vi "CoffeeMachine.vi"() -> ()   [LabVIEW 2020]
uses:
  Typedefs/Operations.ctl
  Typedefs/CoffeeMachineData.ctl
  <vilib>/Utility/config.llb/Config Data RefNum.ctl
  <vilib>/Utility/config.llb/Read Key (I32).vi
  <vilib>/Utility/config.llb/NI_LVConfig.lvlib
panel:
  out "No. of Cups":dbl
  out "Array":i32[](array[numeric])
  out "keys":string[](array[string])
  out "section names":string[](array[string])
  out "Dsipensing":bool
  out "Brewing":bool
  out "Grinding":bool
  out "Heating":bool
  out "Purging":bool
  out "Low Milk":bool
  out "Low Bean":bool
  out "Low Water":bool
  out "Total Cups":dbl
  out "Elapsed Time":i32
  in  "Power":bool
  out "Dispenser":dbl(slide) scale=0.0..60.0
  out "Chamber":dbl(slide) scale=0.0..60.0
  in  "Milk Level":dbl(slide) scale=0.0..100.0
  in  "Bean Level":dbl(slide) scale=0.0..100.0
  in  "Water Level":dbl(slide) scale=0.0..100.0
  in  "Type":u8(knob) scale=0.0..2.0
  in  "1 Carafe":bool
  in  "1 Cup":bool
  in  "Error in (no error)":errorcluster
  out "Error Out":errorcluster
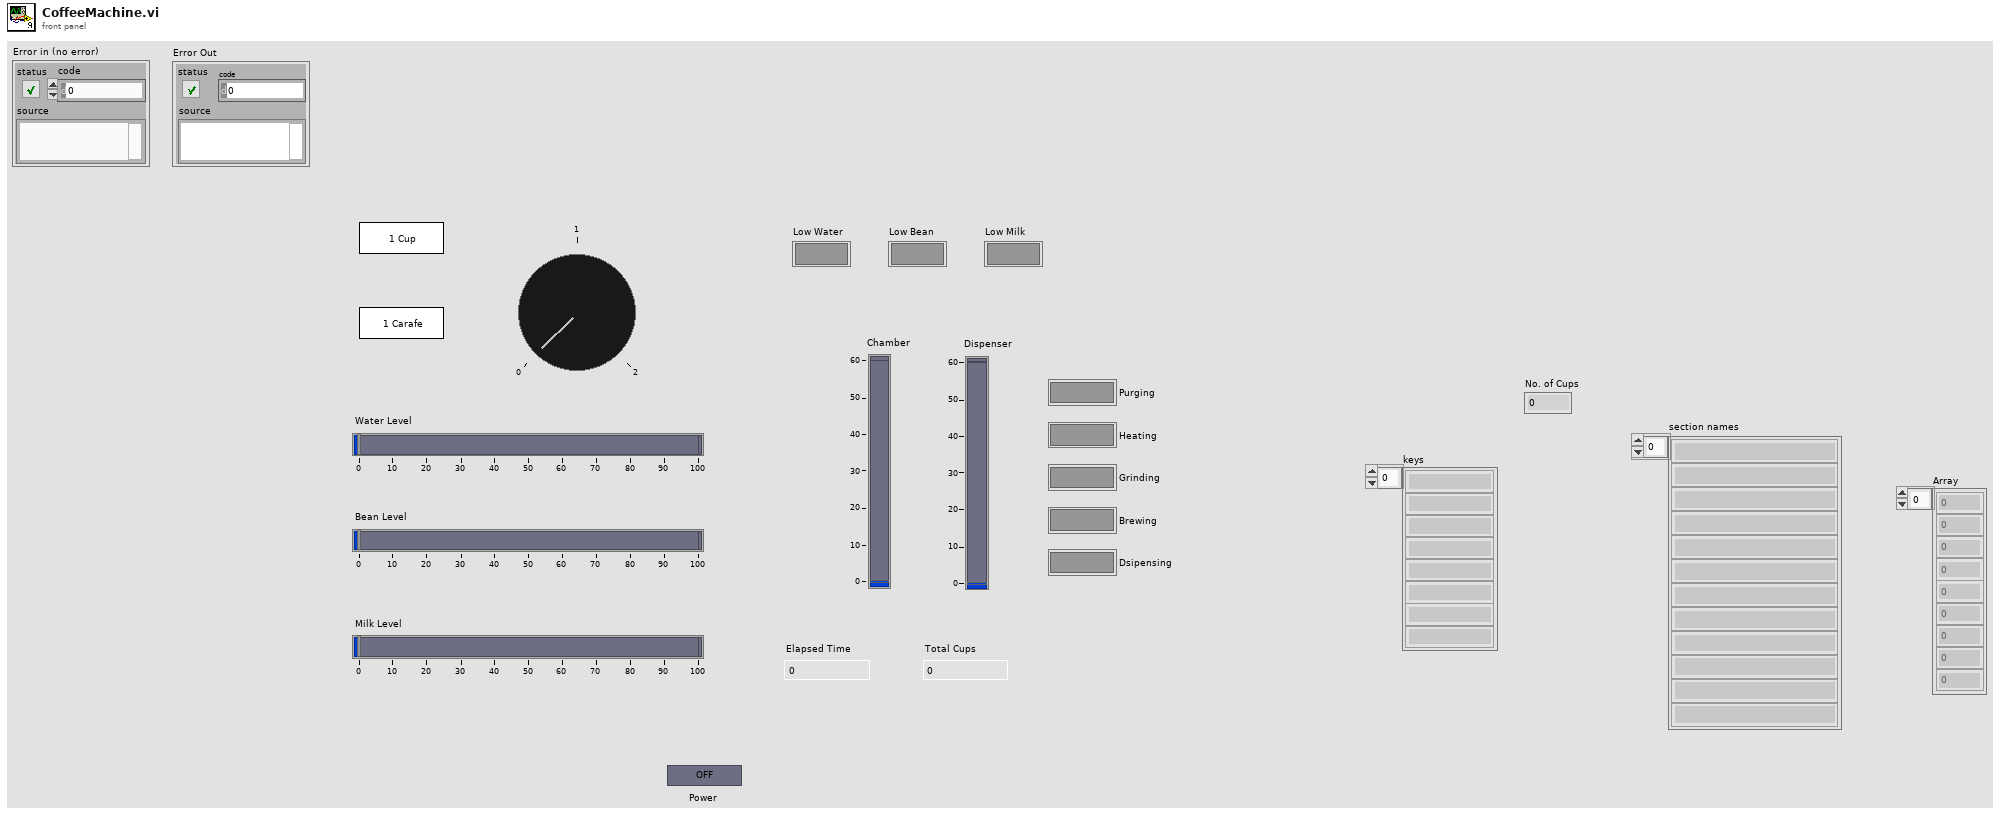
[diagram p1: front panel]
types:
  T1 = typedef "CoffeeMachineData.ctl" = cluster{"Power":bool, "1 Cup":bool, "1 Carafe":bool, "Type":u8, "Water Level":dbl, "Bean Level":dbl, "Milk Level":dbl, "Low Water":bool, "Low Bean":bool, "Low Milk":bool, "Chamber":dbl, "Dispenser":dbl, "Purging":bool, "Heating":bool, "Grinding":bool, "Brewing":bool, "Dispensing":bool, "Elapsed Time":dbl, "Total Cups":dbl, "Start Time":dbl, "File Path":path, "Sufficient Ingredients":bool, "File Reference":T2, "Section Array":string[], "Key Array":string[], "Values Array":i32[], "Section Count":dbl, "Required Section":string, "Type Chosen":bool, "No. of Cups":dbl, "No of Cups Selected":bool}
  T2 = typedef "NI_LVConfig.lvlib/Config Data RefNum.ctl" = refnum<k1>
  T3 = typedef "Operations.ctl" = enum16{"Create Q", "Enqueue 1", "Enqueue N", "Enstack 1", "Dequeue", "Flush Q", "Release Q"}
  T4 = enum8{"Enabled", "Disabled", "Disabled and Grayed Out"}
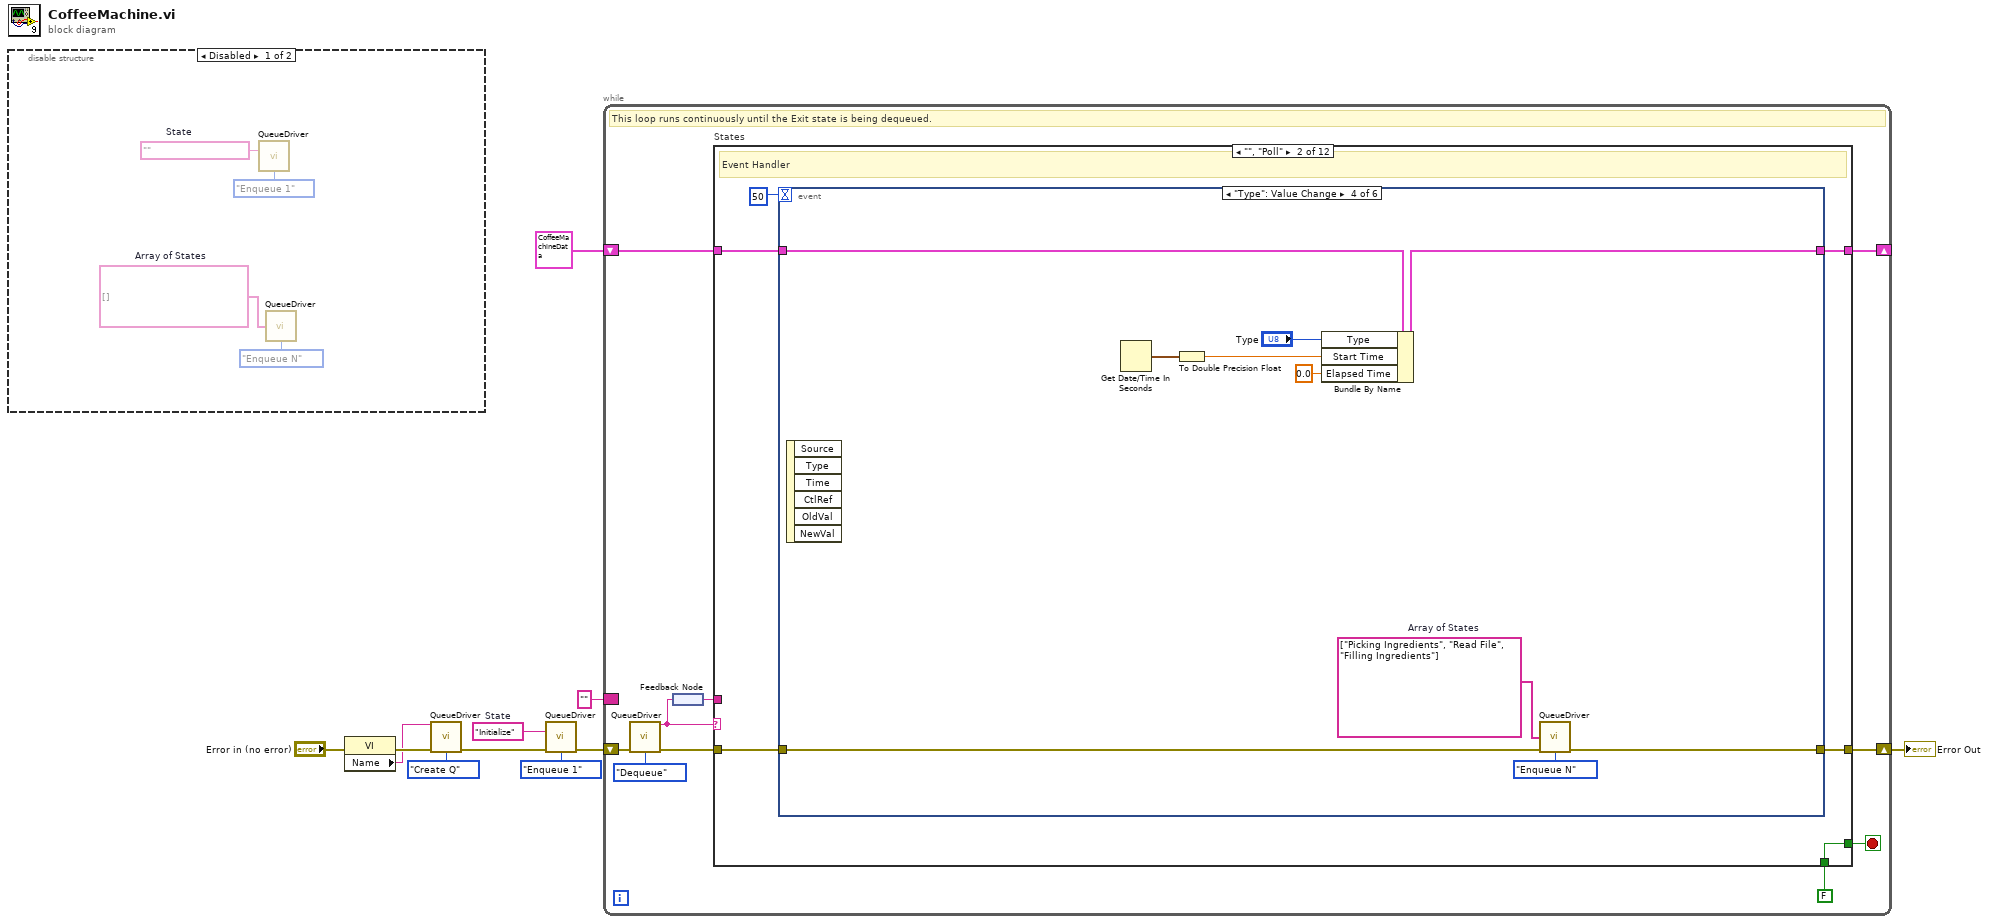
[diagram p0: block diagram]
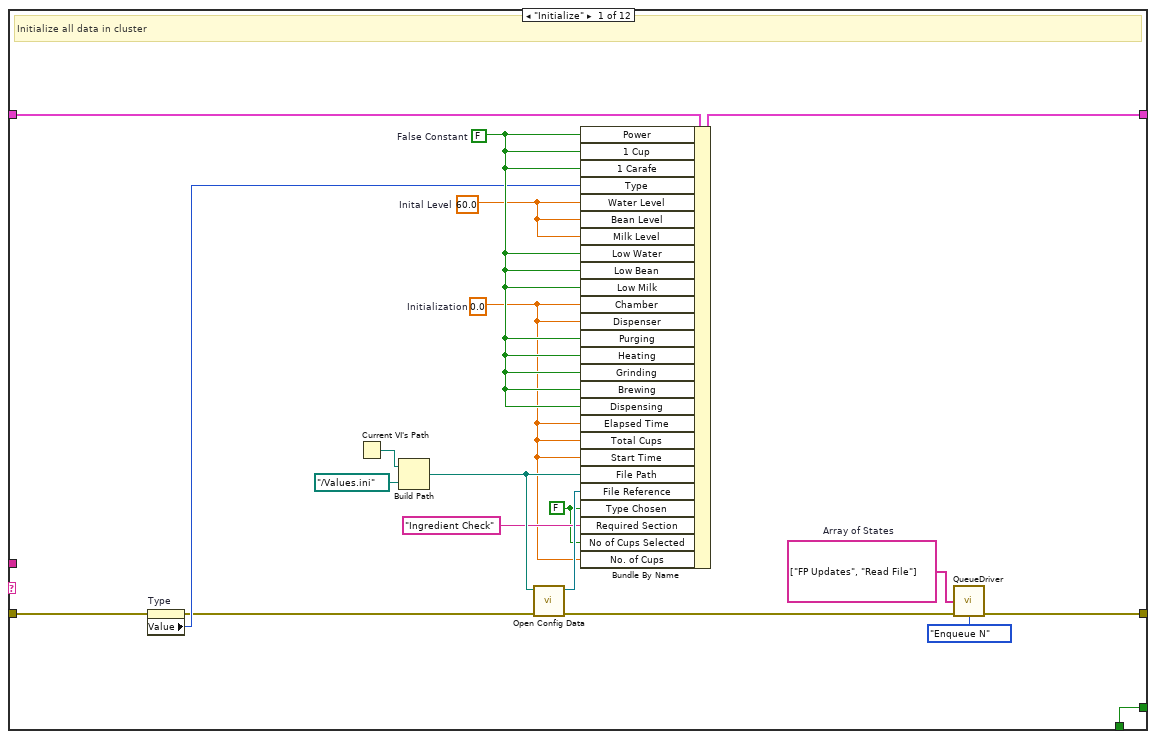
[diagram p3: hidden frame]
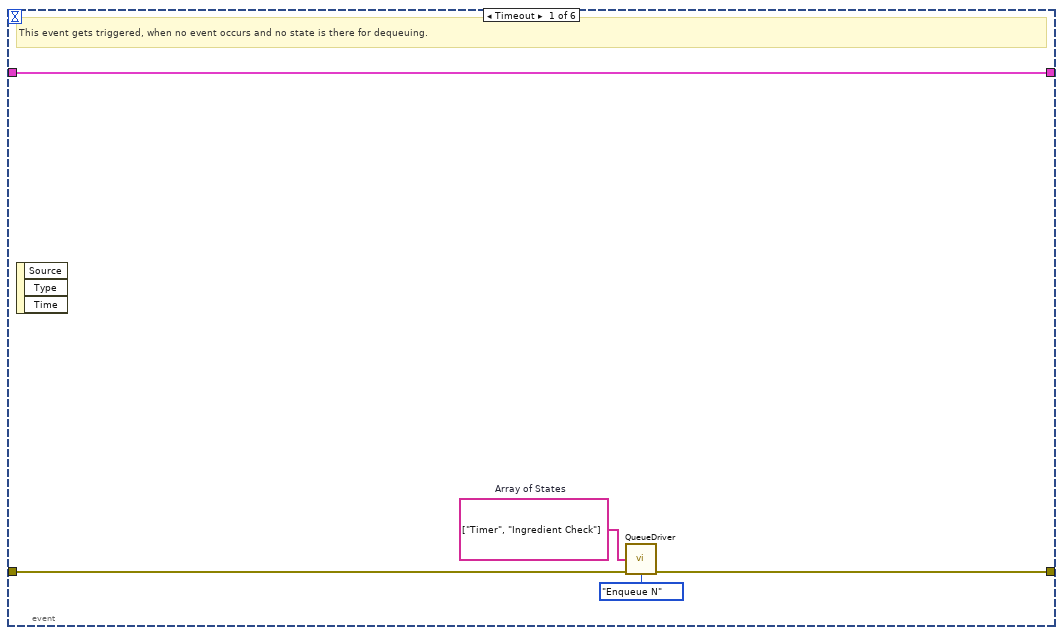
[diagram p4: hidden frame]
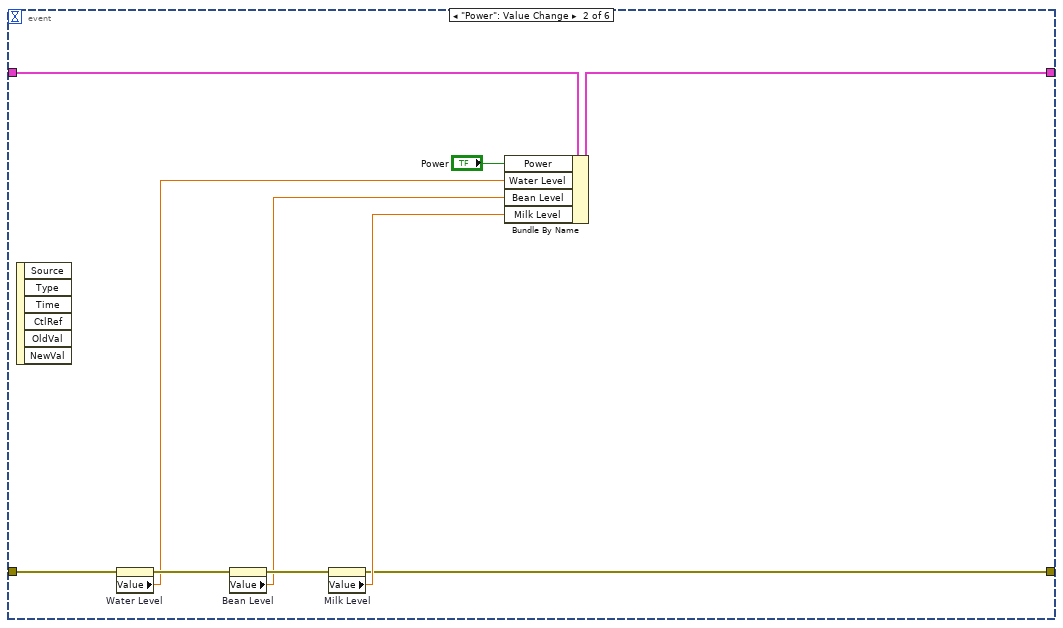
[diagram p5: hidden frame]
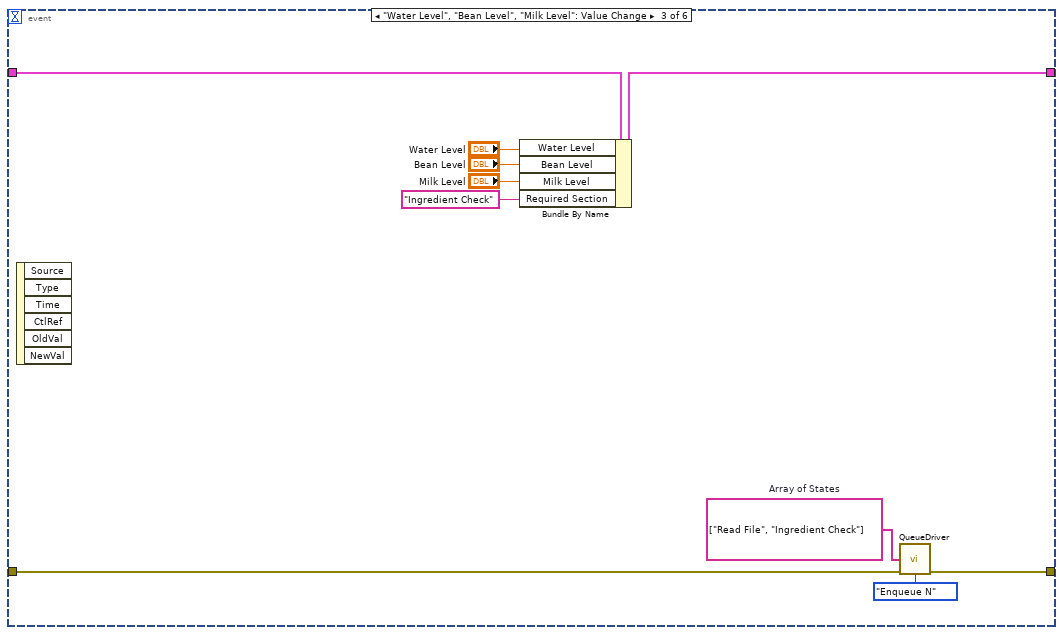
[diagram p6: hidden frame]
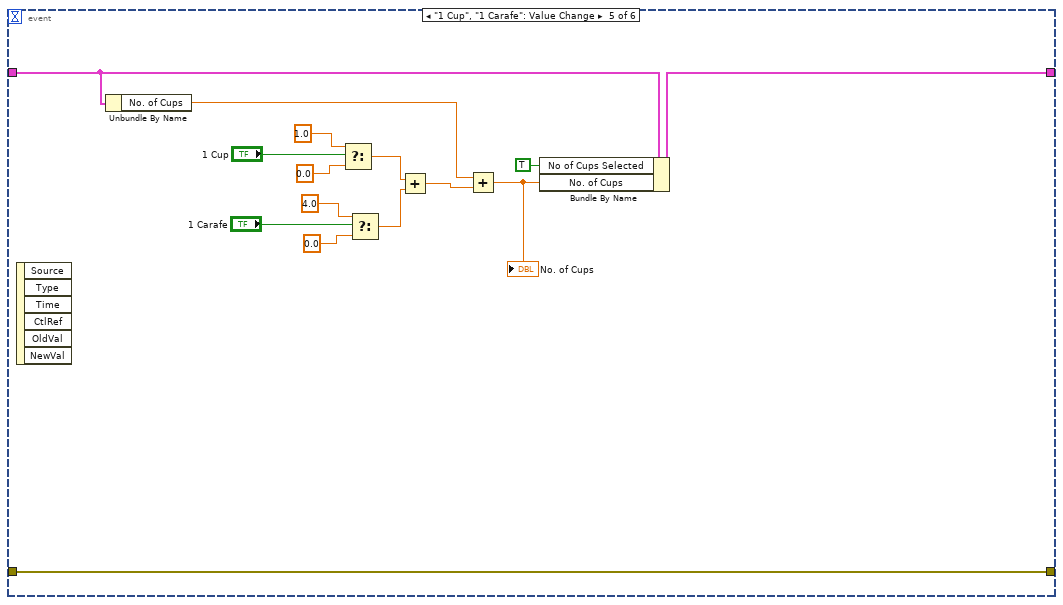
[diagram p7: hidden frame]
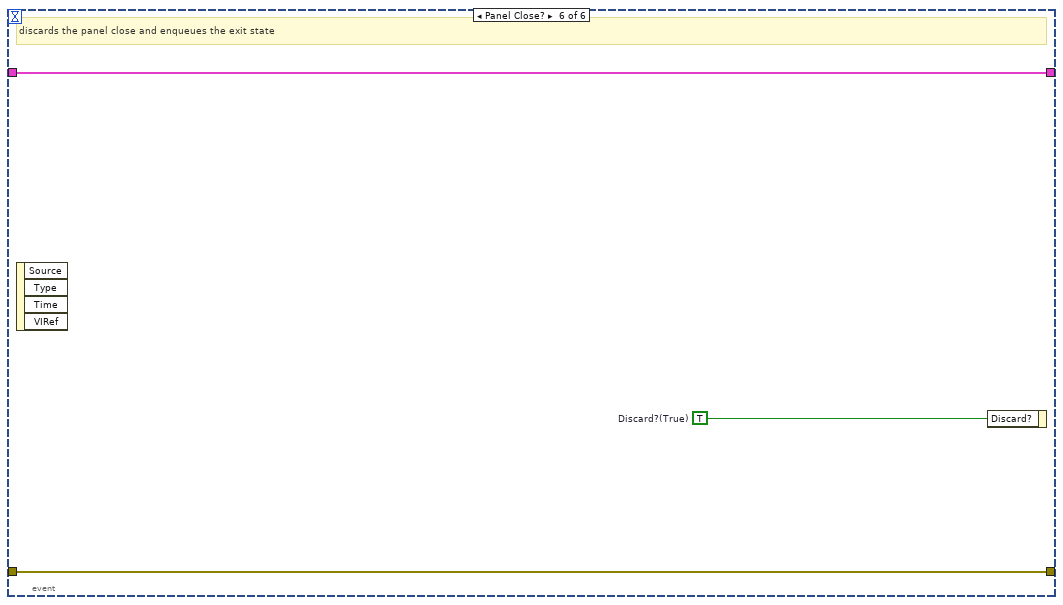
[diagram p8: hidden frame]
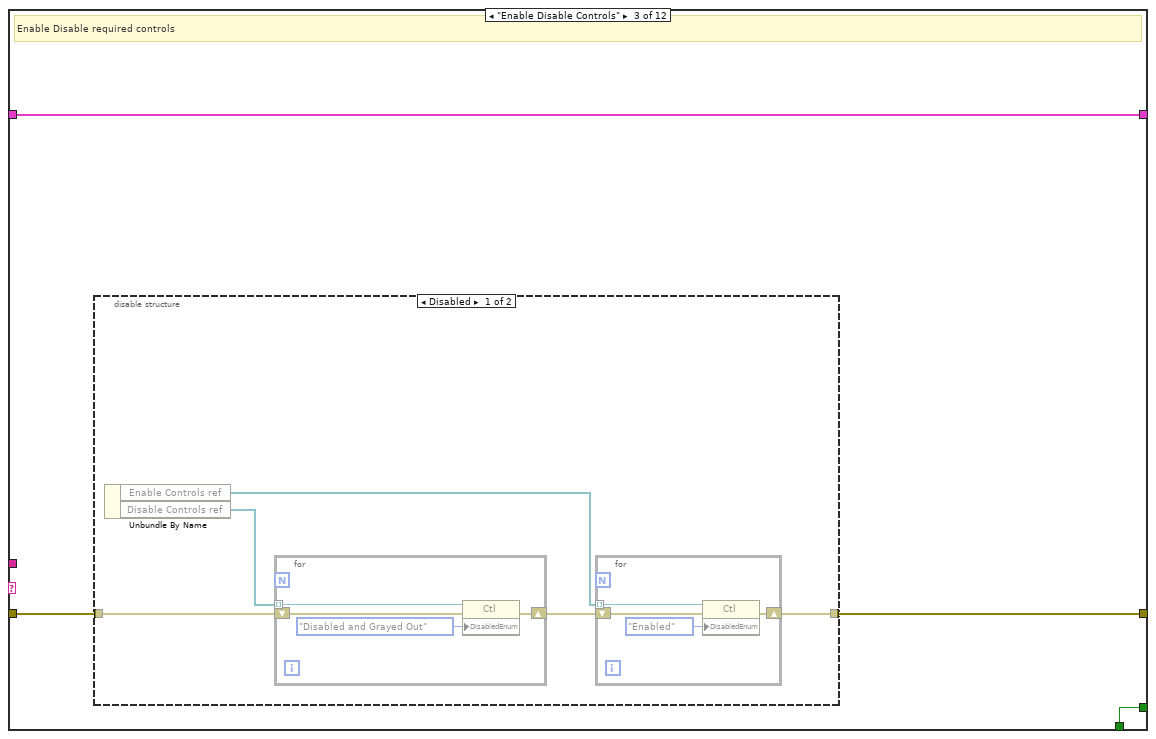
[diagram p9: hidden frame]
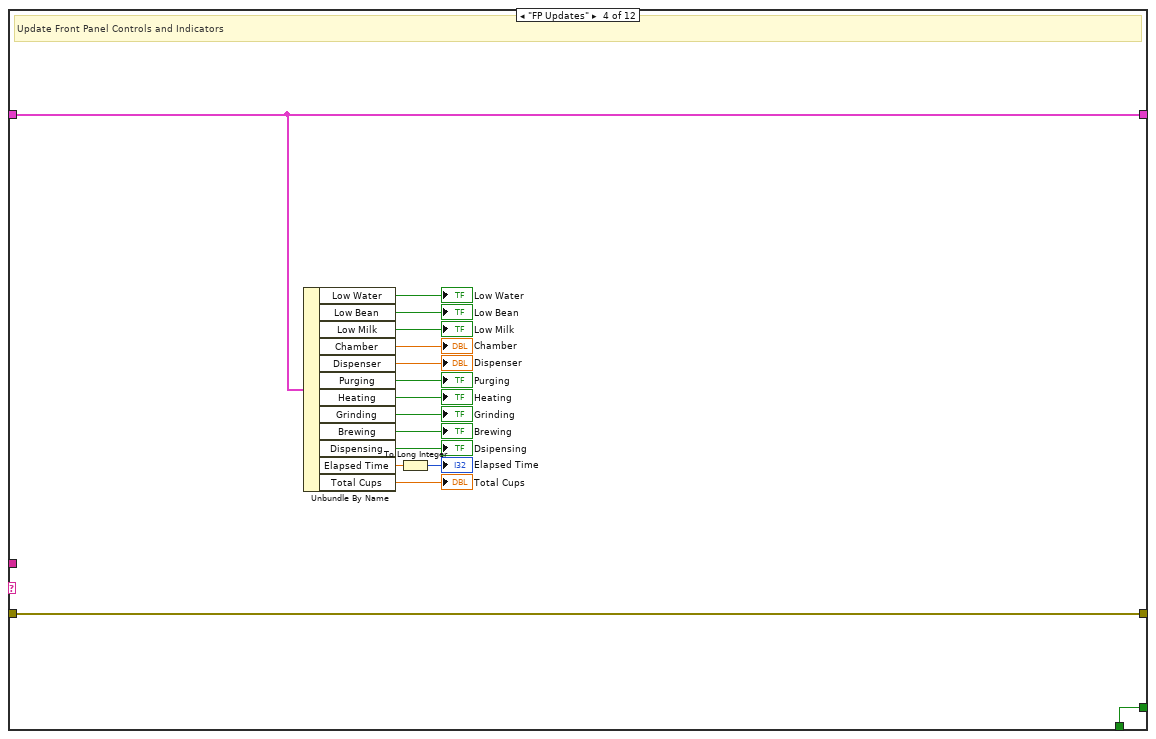
[diagram p11: hidden frame]
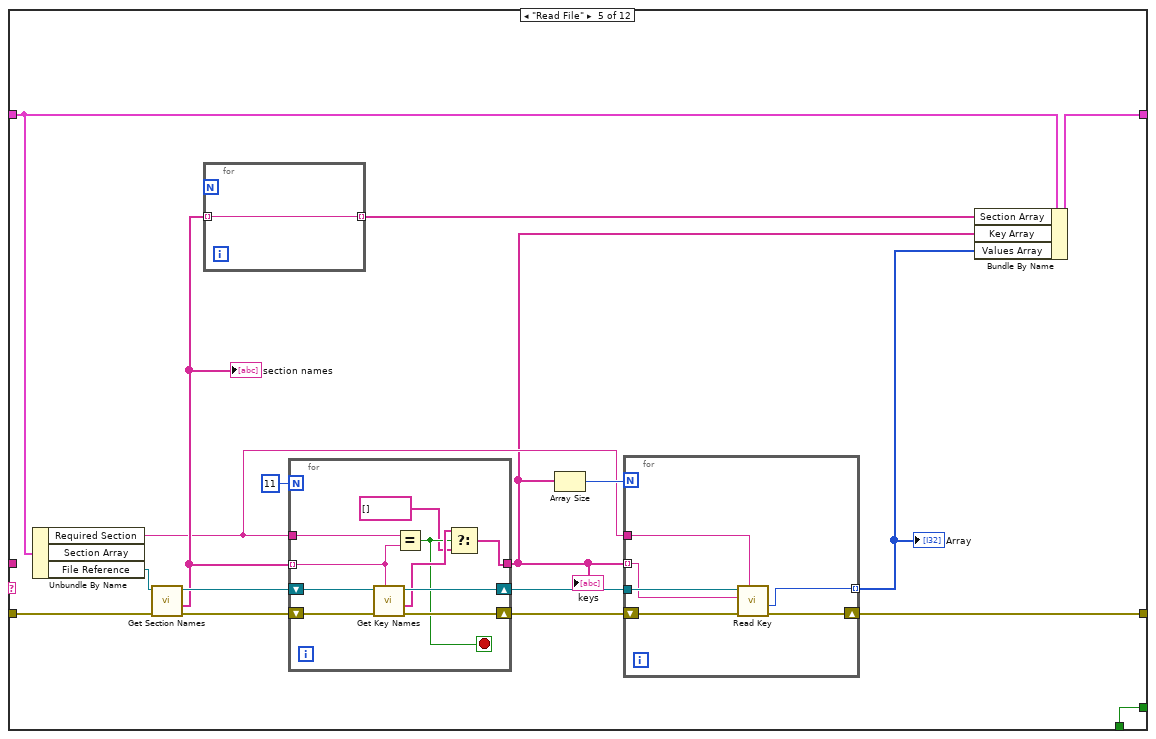
[diagram p12: hidden frame]
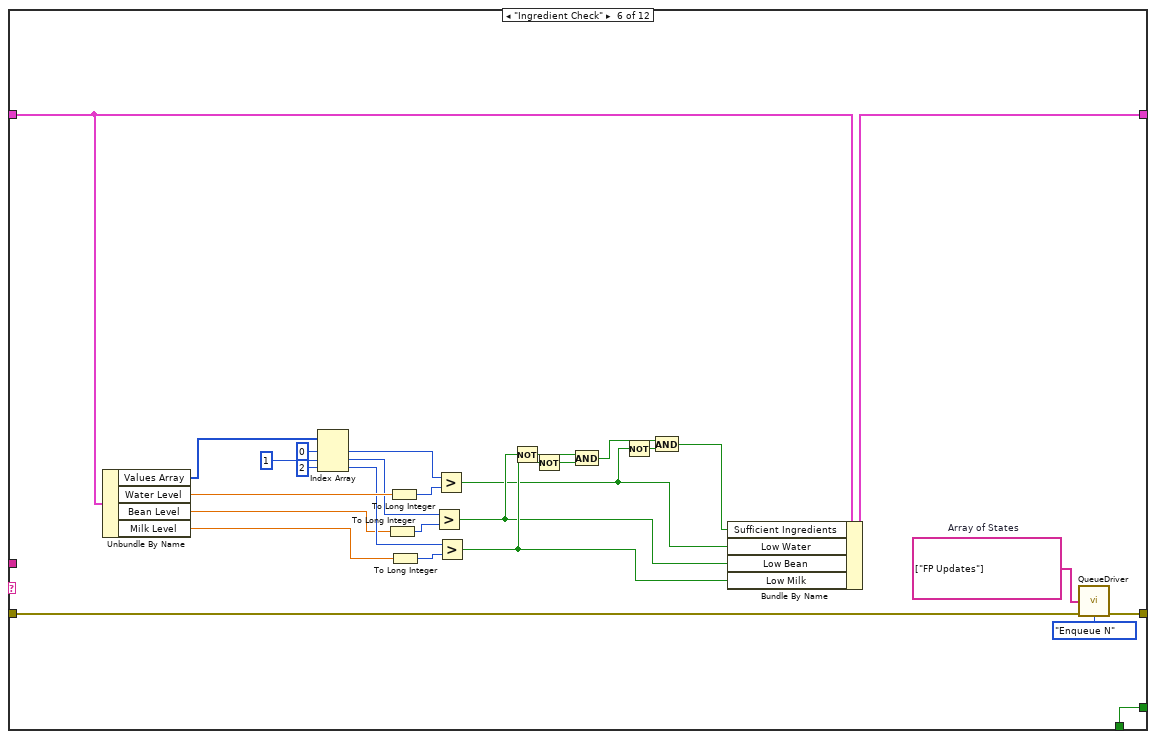
[diagram p13: hidden frame]
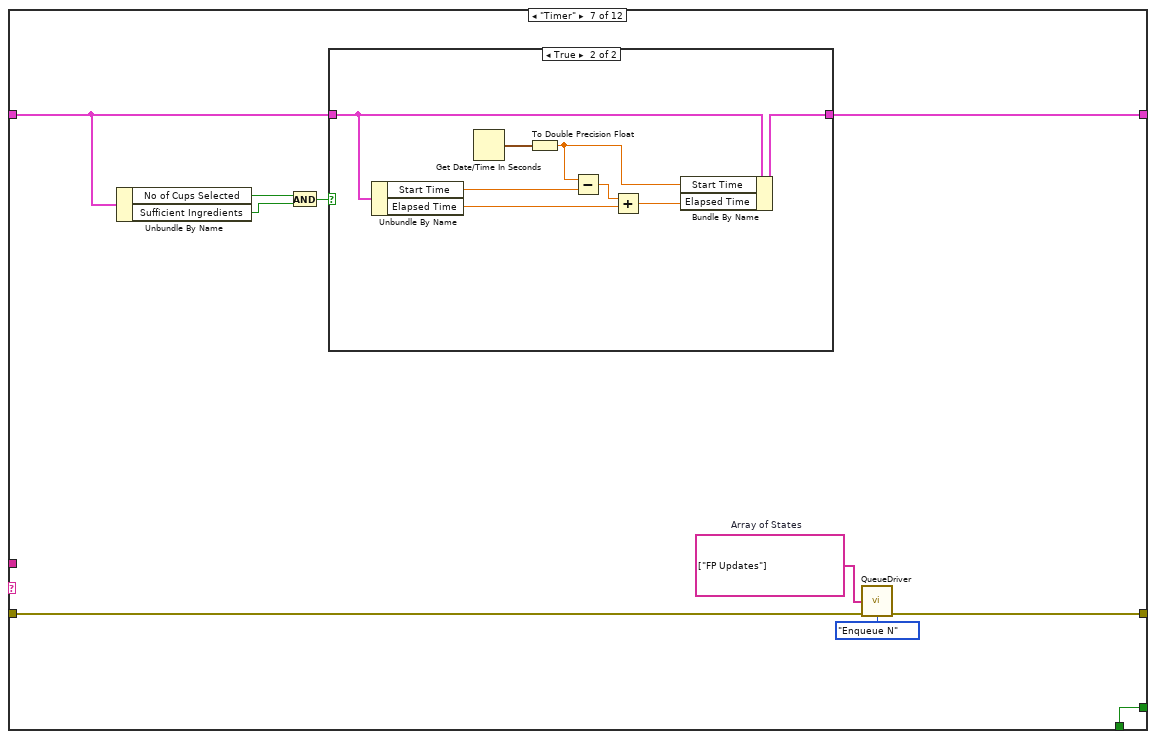
[diagram p14: hidden frame]
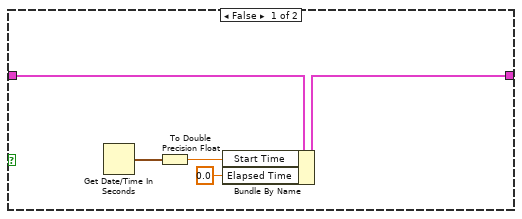
[diagram p15: hidden frame]
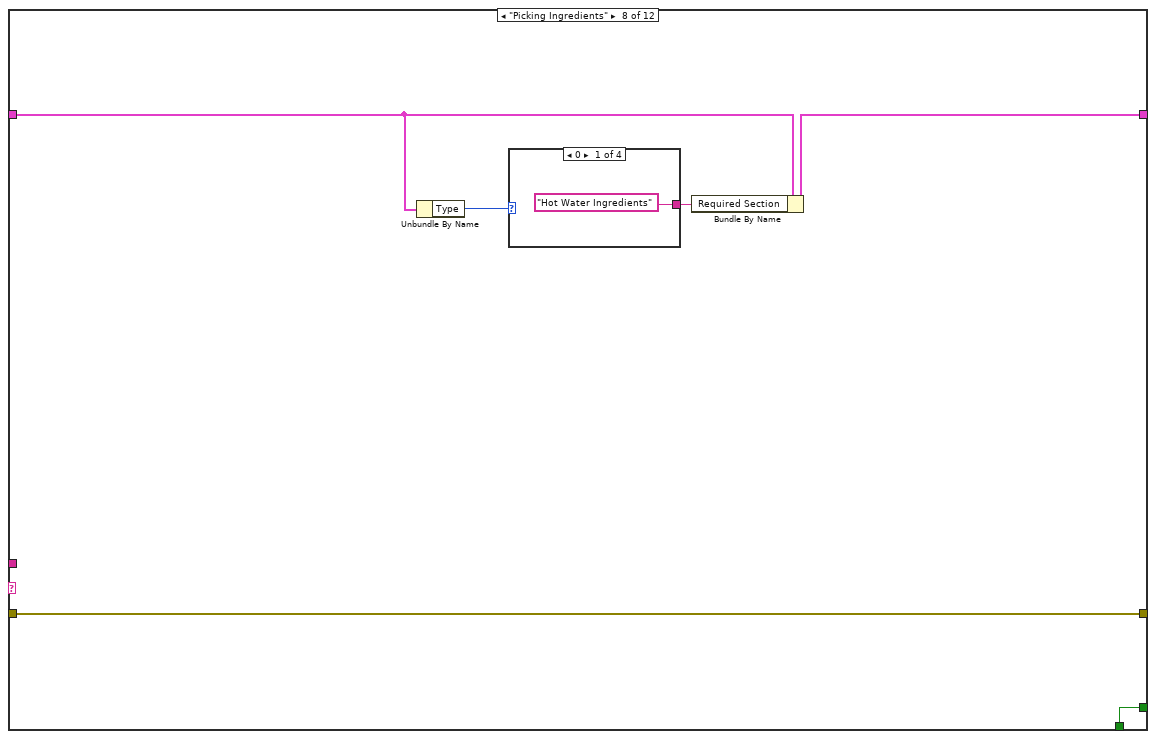
[diagram p16: hidden frame]
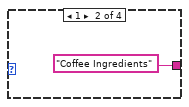
[diagram p17: hidden frame]
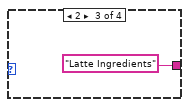
[diagram p18: hidden frame]
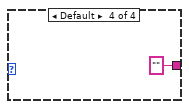
[diagram p19: hidden frame]
diagram:
  w6 = "Initialize"  # State
  n1 = disable-structure shown="Disabled" {
    frame Disabled {
      w12 = string[] []  # Array of States
      w14 = ""  # State
      n2 = call "QueueDriver.vi"("State"=w14, "Operations"=Operations."Enqueue 1" ("Queue Operations")) -> ()  [unwired: 12 in, 2 out]
      n3 = call "QueueDriver.vi"("Array of States"=w12, "Operations"=Operations."Enqueue N" ("Queue Operations")) -> ()  [unwired: 12 in, 2 out]
    }
    frame Enabled {
    }
  }
  n4 = property class="VI"(error in="Error in (no error)") -> (error out=w7:errorcluster, "Name"=w2:string)  [unwired: 1 in, 1 out]
  n5 = call "QueueDriver.vi"("Queue Name"=w2, "error in (no error)"=w7, "Operations"=Operations."Create Q" ("Queue Operations")) -> ("error out"=w3:errorcluster)  [unwired: 11 in, 1 out]
  n6 = call "QueueDriver.vi"("State"=w6, "error in (no error)"=w3, "Operations"=Operations."Enqueue 1" ("Queue Operations")) -> ("error out"=w4:errorcluster)  [unwired: 11 in, 1 out]
  n7 = while {
    border: "" ("States[]") -> [_]
    shift-right: [w24] -> w10
    shift-left: w4 -> [w19]
    shift-right: [w16] -> _
    shift-left: T1 {"Power"=FALSE, "1 Cup"=FALSE, "1 Carafe"=FALSE, "Type"=0, "Water Level"=0.0, "Bean Level"=0.0, "Milk Level"=0.0, "Low Water"=FALSE, "Low Bean"=FALSE, "Low Milk"=FALSE, "Chamber"=0.0, "Dispenser"=0.0, "Purging"=FALSE, "Heating"=FALSE, "Grinding"=FALSE, "Brewing"=FALSE, "Dispensing"=FALSE, "Elapsed Time"=0.0, "Total Cups"=0.0, "Start Time"=0.0, "File Path"=path "", "Sufficient Ingredients"=FALSE, "File Reference"=refnum, "Section Array"=[], "Key Array"=[], "Values Array"=[], "Section Count"=0.0, "Required Section"="", "Type Chosen"=FALSE, "No. of Cups"=0.0, "No of Cups Selected"=FALSE} -> [w17]
    stop <- w23 stop-if-true
    # "This loop runs continuously until the Exit state is being dequeued."
    n8 = call "QueueDriver.vi"("error in (no error)"=w19, "Operations"=Operations."Dequeue" ("Queue Operations")) -> ("Dequeued State"=w18:string, "error out"=w20:errorcluster)  [unwired: 12 in]
    n9 = feedback #1() -> (w25:string)
    n10 = feedback-in #1(w18) -> ()
    n11 = case "States" shown="\"\", \"Poll\"" w18 {
      selector: w18 -> [_ _ _ _ _ _ _ _ _ _ w258 _]
      tunnel: w20 -> [w37 w50 w107 w136 w150 w197 w203 w226 w232 w241 w262 w280]
      tunnel: w25 -> [_ _ _ _ _ _ _ _ _ w240 _ _]
      tunnel: [w29 w49 w106 w136 w147 w192 w202 w226 w232 w237 w259 w278] -> w24
      tunnel: FALSE -> [w44 w48 w105 w135 w153 w191 w206 w227 w234 w236 w257 _]
      tunnel: [w44 w48 w105 w135 w153 w191 w206 w227 w234 w236 w257 TRUE] -> w23
      tunnel: w17 -> [w43 w45 w104 w134 w152 w198 w208 w225 w233 w235 w256 w277]
      tunnel: [w42 w46 w104 w134 w146 w195 w207 w223 w233 w235 w256 w277] -> w16
      frame "Initialize" {
        w27 = FALSE ("Type Chosen")
        w32 = string[] ["FP Updates", "Read File"]  # Array of States
        w26 = 0.0  # Initialization
        w38 = 60.0  # Inital Level
        w39 = FALSE  # False Constant
        # "Initialize all data in cluster"
        n12 = property on="Type" class="Knob (strict)"(error in=w37) -> (error out=w35:errorcluster, "Value"=w36:u8)  [unwired: 1 in, 1 out]
        n13 = Current VI's Path() -> (path=w41:path)
        n14 = Build Path(base path=w41, name or relative path=path "../Values.ini") -> (appended path=w34:path)
        n15 = call <vilib>:"Open Config Data.vi"("error in (no error)"=w35, "configuration file path"=w34) -> ("error out"=w30:errorcluster, "refnum"=w33:T2)  [unwired: 7 in, 1 out]
        n16 = Bundle By Name(cluster=w43, "Power"=w39, "1 Cup"=w39, "1 Carafe"=w39, "Type"=w36, "Water Level"=w38, "Bean Level"=w38, "Milk Level"=w38, "Low Water"=w39, "Low Bean"=w39, "Low Milk"=w39, "Chamber"=w26, "Dispenser"=w26, "Purging"=w39, "Heating"=w39, "Grinding"=w39, "Brewing"=w39, "Dispensing"=w39, "Elapsed Time"=w26, "Total Cups"=w26, "Start Time"=w26, "File Path"=w34, "File Reference"=w33, "Type Chosen"=w27, "Required Section"="Ingredient Check", "No of Cups Selected"=w27, "No. of Cups"=w26) -> (w42:T1)
        n17 = call "QueueDriver.vi"("Array of States"=w32, "error in (no error)"=w30, "Operations"=Operations."Enqueue N" ("Queue Operations")) -> ("error out"=w29:errorcluster)  [unwired: 11 in, 1 out]
      }
      frame "", "Poll" {
        # "Event Handler"
        n18 = event shown="[3] \"Type\": Value Change" {
          selector: _ -> [_ _ _ _ _ _]
          dyn-events: _ -> [_ _ _ _ _ _]
          timeout: 50 -> [_ _ _ _ _ _]
          tunnel: w50 -> [w52 w62 w67 w78 w100 w103]
          tunnel: [w51 w56 w66 w77 w100 w103] -> w49
          tunnel: [w55 w64 w74 w84 w96 w101] -> w46
          tunnel: w45 -> [w55 w65 w75 w85 w89 w101]
          event Timeout {
            w54 = string[] ["Timer", "Ingredient Check"]  # Array of States
            # "This event gets triggered, when no event occurs and no state is there for dequeuing."
            n19 = event-data() -> ()  [unwired: 1 in, 3 out]
            n20 = call "QueueDriver.vi"("Array of States"=w54, "error in (no error)"=w52, "Operations"=Operations."Enqueue N" ("Queue Operations")) -> ("error out"=w51:errorcluster)  [unwired: 11 in, 1 out]
          }
          event "Power": Value Change {
            n21 = event-data() -> ()  [unwired: 1 in, 6 out]
            n22 = property on="Water Level" class="Slide (strict)"(error in=w62) -> (error out=w61:errorcluster, "Value"=w59:dbl)  [unwired: 1 in, 1 out]
            n23 = property on="Bean Level" class="Slide (strict)"(error in=w61) -> (error out=w60:errorcluster, "Value"=w58:dbl)  [unwired: 1 in, 1 out]
            n24 = property on="Milk Level" class="Slide (strict)"(error in=w60) -> (error out=w56:errorcluster, "Value"=w57:dbl)  [unwired: 1 in, 1 out]
            n25 = Bundle By Name(cluster=w65, "Power"="Power", "Water Level"=w59, "Bean Level"=w58, "Milk Level"=w57) -> (w64:T1)
          }
          event "Water Level", "Bean Level", "Milk Level": Value Change {
            w69 = string[] ["Read File", "Ingredient Check"]  # Array of States
            n26 = event-data() -> ()  [unwired: 1 in, 6 out]
            n27 = Bundle By Name(cluster=w75, "Water Level"="Water Level", "Bean Level"="Bean Level", "Milk Level"="Milk Level", "Required Section"="Ingredient Check") -> (w74:T1)
            n28 = call "QueueDriver.vi"("Array of States"=w69, "error in (no error)"=w67, "Operations"=Operations."Enqueue N" ("Queue Operations")) -> ("error out"=w66:errorcluster)  [unwired: 11 in, 1 out]
          }
          event "Type": Value Change {
            w80 = string[] ["Picking Ingredients", "Read File", "Filling Ingredients"]  # Array of States
            n29 = event-data() -> ()  [unwired: 1 in, 6 out]
            n30 = Get Date/Time In Seconds() -> (seconds since 1Jan1904=w82:timestamp)
            n31 = To Double Precision Float(number=w82) -> (double precision float=w81:dbl)
            n32 = Bundle By Name(cluster=w85, "Type"="Type", "Start Time"=w81, "Elapsed Time"=0.0) -> (w84:T1)
            n33 = call "QueueDriver.vi"("Array of States"=w80, "error in (no error)"=w78, "Operations"=Operations."Enqueue N" ("Queue Operations")) -> ("error out"=w77:errorcluster)  [unwired: 11 in, 1 out]
          }
          event "1 Cup", "1 Carafe": Value Change {
            n34 = event-data() -> ()  [unwired: 1 in, 6 out]
            n35 = Unbundle By Name(w89) -> ("No. of Cups"=w88:dbl)
            n36 = Select(t=1.0, s="1 Cup", f=0.0) -> (s? t:f=w91:dbl)
            n37 = Select(t=4.0, s="1 Carafe", f=0.0) -> (s? t:f=w90:dbl)
            n38 = Add(x=w91, y=w90) -> (x+y=w86:dbl)
            n39 = Add(x=w88, y=w86) -> (x+y=w87:dbl)
            "No. of Cups" <- w87
            n40 = Bundle By Name(cluster=w89, "No of Cups Selected"=TRUE, "No. of Cups"=w87) -> (w96:T1)
          }
          event Panel Close? {
            w102 = TRUE  # Discard?(True)
            # "discards the panel close and enqueues the exit state"
            n41 = event-data() -> ()  [unwired: 1 in, 4 out]
            n42 = event-data("Discard?"=w102) -> ()  [unwired: 1 in, 1 out]
          }
        }
      }
      frame "Enable Disable Controls" {
        # "Enable Disable required controls"
        n43 = disable-structure shown="Disabled" {
          disable-tunnel: w107 -> [w112 _]
          disable-tunnel: [w108 _] -> w106
          frame Disabled {
            n44 = Unbundle By Name() -> ("Enable Controls ref"=w109:refnum<vi>[], "Disable Controls ref"=w111:refnum<vi>[])  [unwired: 1 in]
            n45 = for {
              shift-right: [w119] -> w110
              shift-left: w112 -> [w120]
              tunnel: w111 -> [w117] mode=indexing
              n46 = property class="Ctl"(reference=w117, error in=w120, "DisabledEnum"=T4."Disabled and Grayed Out" ("Disabled")) -> (error out=w119:errorcluster)  [unwired: 1 out]
            }
            n47 = for {
              shift-right: [w115] -> w108
              shift-left: w110 -> [w116]
              tunnel: w109 -> [w113] mode=indexing
              n48 = property class="Ctl"(reference=w113, error in=w116, "DisabledEnum"=T4."Enabled" ("Disabled")) -> (error out=w115:errorcluster)  [unwired: 1 out]
            }
          }
          frame Enabled {
          }
        }
      }
      frame "FP Updates" {
        # "Update Front Panel Controls and Indicators"
        n49 = Unbundle By Name(w134) -> ("Low Water"=→"Low Water":bool, "Low Bean"=→"Low Bean":bool, "Low Milk"=→"Low Milk":bool, "Chamber"=→"Chamber":dbl, "Dispenser"=→"Dispenser":dbl, "Purging"=→"Purging":bool, "Heating"=→"Heating":bool, "Grinding"=→"Grinding":bool, "Brewing"=→"Brewing":bool, "Dispensing"=→"Dsipensing":bool, "Elapsed Time"=w123:dbl, "Total Cups"=→"Total Cups":dbl)
        n50 = To Long Integer(number=w123) -> (32bit integer=→"Elapsed Time":i32)
      }
      frame "Read File" {
        n51 = Unbundle By Name(w152) -> ("Required Section"=w139:string, "File Reference"=w151:T2)  [unwired: 1 out]
        n52 = call <vilib>:"Get Section Names.vi"("error in (no error)"=w150, "refnum"=w151) -> ("error out"=w149:errorcluster, "section names"=w142:string[], "refnum out"=w145:T2)  [unwired: 7 in]
        "section names" <- w142
        n53 = for {
          tunnel: w142 -> [w170] mode=indexing
          tunnel: [w170] -> w143 mode=indexing
        }
        n54 = for {
          N: 11 -> [_]
          shift-right: [w168] -> w148
          shift-left: w149 -> [w169]
          shift-right: [w166] -> w144
          shift-left: w145 -> [w167]
          tunnel: w142 -> [w165] mode=indexing
          tunnel: w139 -> [w164]
          tunnel: [w162] -> w137
          stop <- w161 stop-if-true
          n55 = call <vilib>:"Get Key Names.vi"("section"=w165, "error in (no error)"=w169, "refnum"=w167) -> ("error out"=w168:errorcluster, "key names"=w163:string[], "refnum out"=w166:T2)  [unwired: 5 in, 1 out]
          n56 = Equal?(x=w164, y=w165) -> (x = y?=w161:bool)
          n57 = Select(t=w163, s=w161, f=string[] []) -> (s? t:f=w162:string[])
        }
        "keys" <- w137
        n58 = Array Size(array=w137) -> (size(s)=w140:i32)
        n59 = for {
          N: w140 -> [_]
          tunnel: w144 -> [w157]
          shift-right: [w158] -> w147
          shift-left: w148 -> [w159]
          tunnel: w139 -> [w156]
          tunnel: w137 -> [w155] mode=indexing
          tunnel: [w154] -> w138 mode=indexing
          n60 = call-poly <vilib>:"Read Key.vi"("section"=w156, "error in (no error)"=w159, "key"=w155, "refnum"=w157) -> ("error out"=w158:errorcluster, "value"=w154:i32)  [unwired: 4 in, 2 out]
        }
        "Array" <- w138
        n61 = Bundle By Name(cluster=w152, "Section Array"=w143, "Key Array"=w137, "Values Array"=w138) -> (w146:T1)
      }
      frame "Ingredient Check" {
        w194 = string[] ["FP Updates"]  # Array of States
        n62 = Unbundle By Name(w198) -> ("Values Array"=w189:i32[], "Water Level"=w196:dbl, "Bean Level"=w180:dbl, "Milk Level"=w179:dbl)
        n63 = Index Array(array=w189, index #1=0 ("index"), index #2=1 ("index"), index #3=2 ("index")) -> (element #1=w185:i32, element #2=w182:i32, element #3=w181:i32)
        n64 = To Long Integer(number=w180) -> (32bit integer=w183:i32)
        n65 = To Long Integer(number=w196) -> (32bit integer=w190:i32)
        n66 = To Long Integer(number=w179) -> (32bit integer=w184:i32)
        n67 = Greater?(x=w182, y=w183) -> (0:w177:bool)
        n68 = Greater?(x=w185, y=w190) -> (0:w173:bool)
        n69 = Greater?(x=w181, y=w184) -> (0:w178:bool)
        n70 = Not(x=w177) -> (.not. x?=w175:bool)
        n71 = Not(x=w178) -> (.not. x?=w176:bool)
        n72 = And(x=w175, y=w176) -> (x .and. y?=w174:bool)
        n73 = Not(x=w173) -> (.not. x?=w172:bool)
        n74 = And(x=w174, y=w172) -> (x .and. y?=w171:bool)
        n75 = Bundle By Name(cluster=w198, "Sufficient Ingredients"=w171, "Low Water"=w173, "Low Bean"=w177, "Low Milk"=w178) -> (w195:T1)
        n76 = call "QueueDriver.vi"("Array of States"=w194, "error in (no error)"=w197, "Operations"=Operations."Enqueue N" ("Queue Operations")) -> ("error out"=w192:errorcluster)  [unwired: 11 in, 1 out]
      }
      frame "Timer" {
        w205 = string[] ["FP Updates"]  # Array of States
        n77 = Unbundle By Name(w208) -> ("No of Cups Selected"=w201:bool, "Sufficient Ingredients"=w199:bool)
        n78 = And(x=w201, y=w199) -> (x .and. y?=w200:bool)
        n79 = case shown="True" w200 {
          tunnel: w208 -> [w213 w221]
          tunnel: [w212 w217] -> w207
          frame False {
            n80 = Get Date/Time In Seconds() -> (seconds since 1Jan1904=w210:timestamp)
            n81 = To Double Precision Float(number=w210) -> (double precision float=w209:dbl)
            n82 = Bundle By Name(cluster=w213, "Start Time"=w209, "Elapsed Time"=0.0) -> (w212:T1)
          }
          frame True {
            n83 = Unbundle By Name(w221) -> ("Start Time"=w219:dbl, "Elapsed Time"=w218:dbl)
            n84 = Get Date/Time In Seconds() -> (seconds since 1Jan1904=w220:timestamp)
            n85 = To Double Precision Float(number=w220) -> (double precision float=w214:dbl)
            n86 = Subtract(x=w214, y=w219) -> (x-y=w215:dbl)
            n87 = Add(x=w215, y=w218) -> (x+y=w216:dbl)
            n88 = Bundle By Name(cluster=w221, "Start Time"=w214, "Elapsed Time"=w216) -> (w217:T1)
          }
        }
        n89 = call "QueueDriver.vi"("Array of States"=w205, "error in (no error)"=w203, "Operations"=Operations."Enqueue N" ("Queue Operations")) -> ("error out"=w202:errorcluster)  [unwired: 11 in, 1 out]
      }
      frame "Picking Ingredients" {
        n90 = Unbundle By Name(w225) -> ("Type"=w224:u8)
        n91 = case shown="0" w224 {
          tunnel: ["Hot Water Ingredients" ("Required Section") "Coffee Ingredients" ("Required Section") "Latte Ingredients" ("Required Section") "" ("Required Section")] -> w222
          frame 0 {
          }
          frame 1 {
          }
          frame 2 {
          }
          frame Default {
          }
        }
        n92 = Bundle By Name(cluster=w225, "Required Section"=w222) -> (w223:T1)
      }
      frame "Filling Ingredients" {
      }
      frame "Error" {
        # "Handle Errors"
        n93 = Unbundle By Name(w241) -> ("code"=w246:i32, "source"=w245:string)
        n94 = call <vilib>:"Clear Errors.vi"("error in (no error)"=w241, "specific error code to clear (0: all)"=w246) -> ("error out"=w248:errorcluster)  [unwired: 4 in, 1 out]
        n95 = Format Into String(format string="Error occurred in state \"%s\"!!\nError Code: %d\nError Source: %s\n\nDo you wish to continue?", error in=w248, w240, w246, w245) -> (resulting string=w244:string, error out=w238:errorcluster)  [unwired: 1 in]
        n96 = Two Button Dialog(message=w244, 1:"Exit" ("F button name (\"Cancel\")"), 2:"Continue" ("T button name (\"OK\")")) -> (T button?=w239:bool)
        n97 = case "Continue?" shown="False" w239 {
          tunnel: w238 -> [w250 w255]
          tunnel: [w249 w255] -> w237
          frame False {
            w253 = "Exit"  # State
            # "Exit"
            n98 = call "QueueDriver.vi"("error in (no error)"=w250, "Operations"=Operations."Flush Q" ("Queue Operations")) -> ("error out"=w251:errorcluster)  [unwired: 12 in, 1 out]
            n99 = call "QueueDriver.vi"("State"=w253, "error in (no error)"=w251, "Operations"=Operations."Enqueue 1" ("Queue Operations")) -> ("error out"=w249:errorcluster)  [unwired: 11 in, 1 out]
          }
          frame True {
            # "Continue"
          }
        }
      }
      frame "Developer Error", Default {
        # "You can remove this case after development, and make \"Poll\" as Default case"
        # "Handle Errors"
        n100 = Unbundle By Name(w262) -> ("code"=w267:i32, "source"=w266:string)
        n101 = call <vilib>:"Clear Errors.vi"("error in (no error)"=w262, "specific error code to clear (0: all)"=w267) -> ("error out"=w269:errorcluster)  [unwired: 4 in, 1 out]
        n102 = Format Into String(format string="DEVELOPER ERROR\nState \"%s\" not found!!\nError Code: %d\nError Source: %s\n\nDo you wish to continue?", error in=w269, w258, w267, w266) -> (resulting string=w265:string, error out=w260:errorcluster)  [unwired: 1 in]
        n103 = Two Button Dialog(message=w265, 1:"Exit" ("F button name (\"Cancel\")"), 2:"Continue" ("T button name (\"OK\")")) -> (T button?=w261:bool)
        n104 = case "Continue?" shown="False" w261 {
          tunnel: w260 -> [w274 w276]
          tunnel: [w270 w276] -> w259
          frame False {
            w273 = "Exit"  # State
            # "Exit"
            n105 = call "QueueDriver.vi"("error in (no error)"=w274, "Operations"=Operations."Flush Q" ("Queue Operations")) -> ("error out"=w271:errorcluster)  [unwired: 12 in, 1 out]
            n106 = call "QueueDriver.vi"("State"=w273, "error in (no error)"=w271, "Operations"=Operations."Enqueue 1" ("Queue Operations")) -> ("error out"=w270:errorcluster)  [unwired: 11 in, 1 out]
          }
          frame True {
            # "Continue"
          }
        }
      }
      frame "Exit" {
        # "Exit the State Machine"
        n107 = call "QueueDriver.vi"("error in (no error)"=w280, "Operations"=Operations."Flush Q" ("Queue Operations")) -> ("error out"=w279:errorcluster)  [unwired: 12 in, 1 out]
        n108 = call "QueueDriver.vi"("error in (no error)"=w279, "Operations"=Operations."Release Q" ("Queue Operations")) -> ("error out"=w278:errorcluster)  [unwired: 12 in, 1 out]
      }
    }
  }
  "Error Out" <- w10
